vi "synesthesia-simulator.vi"() -> ()   [LabVIEW 2018]
uses:
  <vilib>/sound2/lvsound2.llb/Sampling Mode.ctl
  <vilib>/sound2/lvsound2.llb/Sound Data Format.ctl
  <vilib>/sound2/lvsound2.llb/Sound Input Read (DBL).vi
  <vilib>/measure/matone.llb/Extract Single Tone Information 1 Chan.vi
  <vilib>/express/express analysis/Spectral/Block/exnSpectralBlock spectral measurements peak poly.vi
  <vilib>/express/express analysis/Spectral/Block/exnSpectralBlock spectral measurements peak WFM.vi
  <vilib>/express/express analysis/Spectral/XNode/ExpressSpectralMeasurementsBlockNode.xnode
  <vilib>/measure/NI_MAPro.lvlib
panel:
  out "Wavelength":dbl
  out "Color":u32(colorbox)=4980812
  out "Out Of Range":bool
  in  "stop":bool
  out "Frequency Power Spectrum":cluster{"f0":dbl, "df":dbl, "magnitude":dbl[]}(graph)
  out "Tiime domain signal":waveform(dbl)(graph)
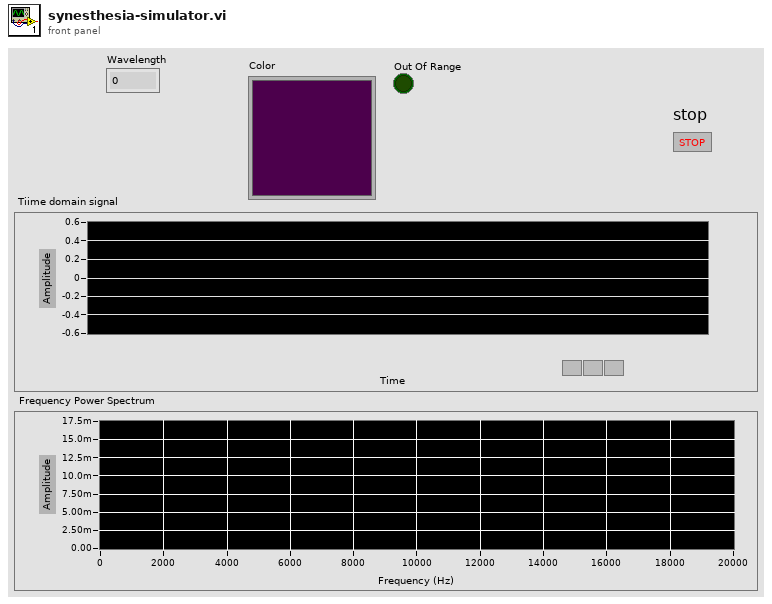
[diagram p1: front panel]
types:
  T1 = typedef "Sound Data Format.ctl" = cluster{"sample rate (S/s)":dbl, "number of channels":i32, "bits per sample":i32}
  T2 = typedef "Sampling Mode.ctl" = i32
  T3 = typedef "Sound Input Task ID.ctl" = u32
  T4 = cluster{"averaging mode":u16, "weighting mode":u16, "number of averages":u32}
  T5 = cluster{"dB On (F)":bool, "unwrap phase (F)":bool, "convert to degree (F)":bool}
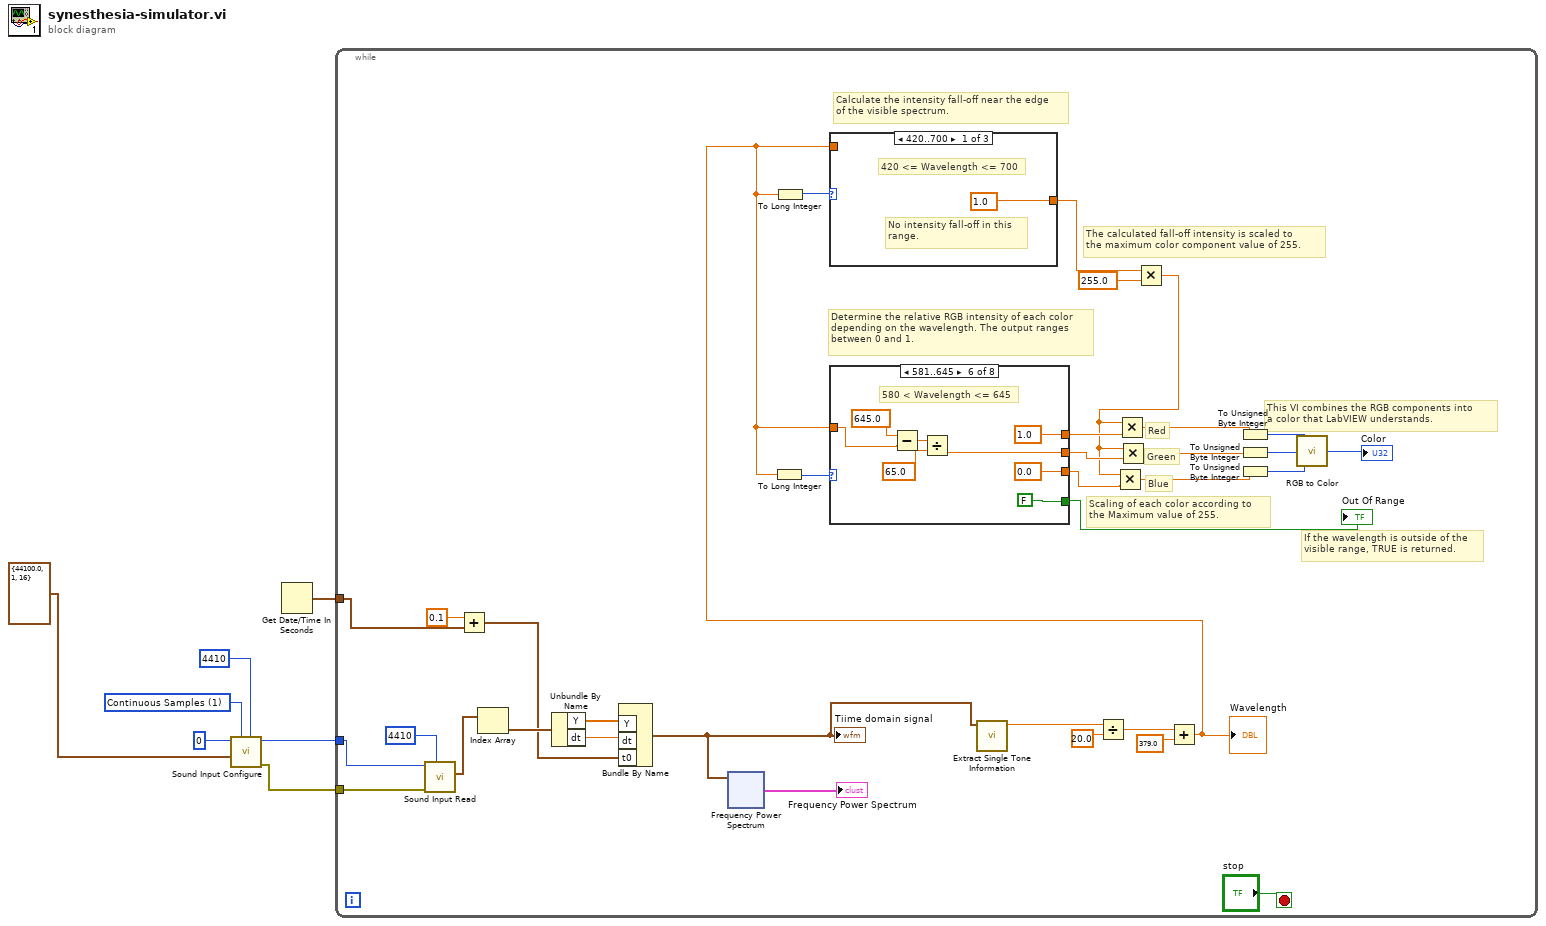
[diagram p0: block diagram]
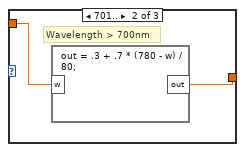
[diagram p2: hidden frame]
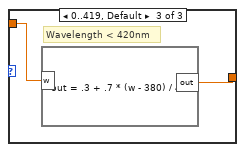
[diagram p3: hidden frame]
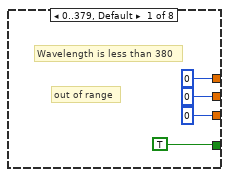
[diagram p4: hidden frame]
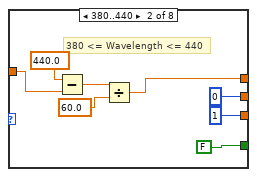
[diagram p5: hidden frame]
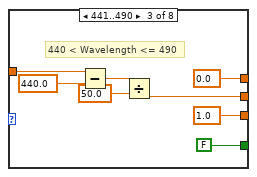
[diagram p6: hidden frame]
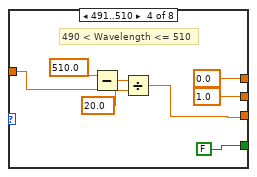
[diagram p7: hidden frame]
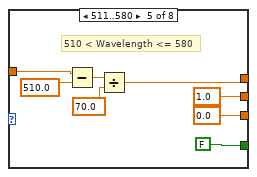
[diagram p8: hidden frame]
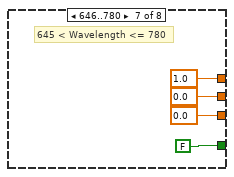
[diagram p9: hidden frame]
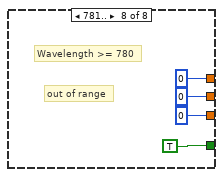
[diagram p10: hidden frame]
diagram:
  w6 = T2 1 items=["Finite Samples", "Continuous Samples"] ("sample mode")
  n1 = call <vilib>:"Sound Input Configure.vi"("number of samples/ch"=4410 ("Number of Samples"), "sample mode"=w6, "sound format"=T1 {"sample rate (S/s)"=44100.0, "number of channels"=1, "bits per sample"=16}, "device ID"=0) -> ("error out"=w4:errorcluster, "task ID"=w3:T3)  [unwired: 6 in]
  n2 = Get Date/Time In Seconds() -> (seconds since 1Jan1904=w2:timestamp)
  n3 = while {
    tunnel: w4 -> [w41]
    tunnel: w3 -> [w40]
    tunnel: w2 -> [w34]
    stop <- "stop" stop-if-true
    # "This VI combines the RGB components into\na color that LabVIEW understands."
    # "If the wavelength is outside of the\nvisible range, TRUE is returned."
    # "Blue"
    # "Green"
    # "Red"
    # "The calculated fall-off intensity is scaled to\nthe maximum color component value of 255."
    # "Scaling of each color according to\nthe Maximum value of 255."
    # "Determine the relative RGB intensity of each color\ndepending on the wavelength. The output ranges\nbetween 0 and 1."
    # "Calculate the intensity fall-off near the edge\nof the visible spectrum."
    n4 = call-poly <vilib>:"Sound Input Read.vi"("number of samples/ch"=4410, "error in (no error)"=w41, "task ID"=w40) -> ("data"=w38:waveform(dbl)[])  [unwired: 6 in, 2 out]
    n5 = Add(x=0.1, y=w34) -> (x+y=w32:timestamp)
    n6 = Index Array(array=w38) -> (element=w37:waveform(dbl))  [unwired: 1 in]
    n7 = Unbundle By Name(w37) -> ("Y"=w36:dbl[], "dt"=w35:dbl)
    n8 = Bundle By Name("Y"=w36, "dt"=w35, "t0"=w32) -> (w8:waveform(dbl))  [unwired: 1 in]
    "Tiime domain signal" <- w8
    n9 = xnode "Frequency Power Spectrum"("Signals"=w8) -> ("FFT - (Peak)"=→"Frequency Power Spectrum":cluster{"f0":dbl, "df":dbl, "magnitude":dbl[]})  [unwired: 1 in, 2 out]
    n10 = call-poly <vilib>:"Extract Single Tone Information.vi"("time signal in"=w8) -> ("detected frequency"=w9:dbl)  [unwired: 5 in, 5 out]
    n11 = Divide(x=w9, y=20.0) -> (x/y=w12:dbl)
    n12 = Add(x=w12, y=379.0) -> (x+y=w10:dbl)
    "Wavelength" <- w10
    n13 = To Long Integer(number=w10) -> (32bit integer=w15:i32)
    n14 = To Long Integer(number=w10) -> (32bit integer=w14:i32)
    n15 = case shown="420..700" w14 {
      tunnel: w10 -> [_ w44 w45]
      tunnel: [1.0 w43 w46] -> w24
      frame 420..700 {
        # "No intensity fall-off in this\nrange."
        # "420 <= Wavelength <= 700"
      }
      frame 701.. {
        # "Wavelength > 700nm"
        n16 = formula code="out = .3 + .7 * (780 - w) / 80;"("w"=w44) -> ("out"=w43:dbl)
      }
      frame 0..419, Default {
        # "Wavelength < 420nm"
        n17 = formula code="out = .3 + .7 * (w - 380) / 40;"("w"=w45) -> ("out"=w46:dbl)
      }
    }
    n18 = case shown="581..645" w15 {
      tunnel: w10 -> [_ w55 w65 w72 w81 w89 _ _]
      tunnel: [u32 0 w51 0.0 0.0 w77 1.0 1.0 u32 0] -> w22
      tunnel: [u32 0 u32 0 w61 1.0 1.0 w85 0.0 u32 0] -> w21
      tunnel: [u32 0 u32 1 1.0 w69 0.0 0.0 0.0 u32 0] -> w20
      tunnel: [TRUE FALSE FALSE FALSE FALSE FALSE FALSE TRUE] -> w29
      frame 0..379, Default {
        # "out of range"
        # "Wavelength is less than 380"
      }
      frame 380..440 {
        # "380 <= Wavelength <= 440"
        n19 = Subtract(x=440.0, y=w55) -> (x-y=w53:dbl)
        n20 = Divide(x=w53, y=60.0) -> (x/y=w51:dbl)
      }
      frame 441..490 {
        # "440 < Wavelength <= 490"
        n21 = Subtract(x=w65, y=440.0) -> (x-y=w63:dbl)
        n22 = Divide(x=w63, y=50.0) -> (x/y=w61:dbl)
      }
      frame 491..510 {
        # "490 < Wavelength <= 510"
        n23 = Subtract(x=510.0, y=w72) -> (x-y=w71:dbl)
        n24 = Divide(x=w71, y=20.0) -> (x/y=w69:dbl)
      }
      frame 511..580 {
        # "510 < Wavelength <= 580"
        n25 = Subtract(x=w81, y=510.0) -> (x-y=w79:dbl)
        n26 = Divide(x=w79, y=70.0) -> (x/y=w77:dbl)
      }
      frame 581..645 {
        # "580 < Wavelength <= 645"
        n27 = Subtract(x=645.0, y=w89) -> (x-y=w87:dbl)
        n28 = Divide(x=w87, y=65.0) -> (x/y=w85:dbl)
      }
      frame 646..780 {
        # "645 < Wavelength <= 780"
      }
      frame 781.. {
        # "out of range"
        # "Wavelength >= 780"
      }
    }
    "Out Of Range" <- w29
    n29 = Multiply(x=w24, y=255.0) -> (x*y=w16:dbl)
    n30 = Multiply(x=w16, y=w20) -> (x*y=w17:dbl)
    n31 = Multiply(x=w16, y=w22) -> (x*y=w19:dbl)
    n32 = Multiply(x=w16, y=w21) -> (x*y=w18:dbl)
    n33 = To Unsigned Byte Integer(number=w19) -> (unsigned 8bit integer=w27:u8)
    n34 = To Unsigned Byte Integer(number=w18) -> (unsigned 8bit integer=w26:u8)
    n35 = To Unsigned Byte Integer(number=w17) -> (unsigned 8bit integer=w25:u8)
    n36 = call "RGB to Color.vi"("B"=w25, "G"=w26, "R"=w27) -> ("Color"=→"Color":u32)
  }
